vi "M_alpha_beta_2 (SubVI).vi"(4 "i":i32, 6 "Fe_data":dbl[](array[numeric]), 7 "FE [N]":dbl[](array[numeric]), 8 "Vehicle Parameters":T1, 10 "Data":dbl[][](array[numeric]), 11 "cluster":T3) -> (0 "output cluster":T2, 2 "M_beta":dbl, 3 "M_alpha":dbl)   [LabVIEW 2017]
uses:
  <vilib>/Analysis/_algsub.llb/Vector Norm Type.ctl
  <vilib>/Analysis/_algsub.llb/Real Vector Norm.vi
  <vilib>/Analysis/NI_AALPro.lvlib
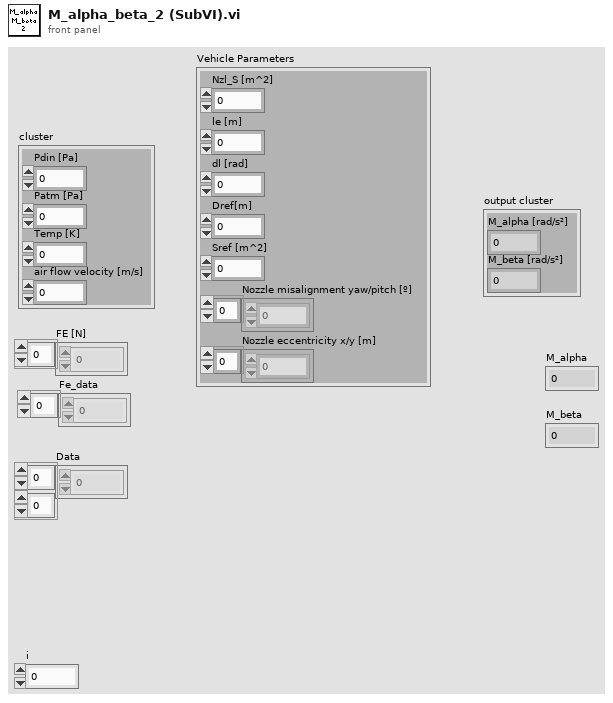
[diagram p1: front panel]
types:
  T1 = cluster{"Nzl_S [m^2]":dbl, "le [m]":dbl, "dl [rad]":dbl, "Dref[m]":dbl, "Sref [m^2]":dbl, "Nozzle misalignment yaw/pitch [º]":dbl[], "Nozzle eccentricity x/y [m]":dbl[]}
  T2 = cluster{"M_alpha [rad/s²]":dbl, "M_beta [rad/s²]":dbl}
  T3 = cluster{"Pdin [Pa]":dbl, "Patm [Pa]":dbl, "Temp [K]":dbl, "air flow velocity [m/s]":dbl}
  T4 = typedef "NI_AALPro.lvlib/Vector Norm Type.ctl" = u16
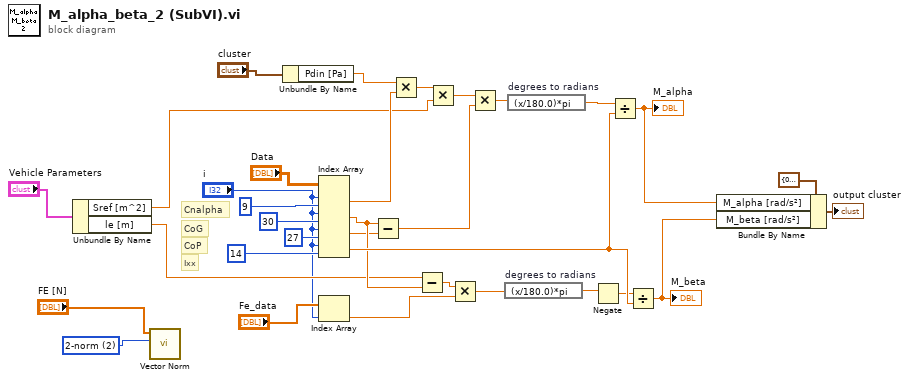
[diagram p0: block diagram]
diagram:
  w26 = T4 2 items=["1-norm"=1, "2-norm"=2, "Inf-norm"=3, "-Inf-norm"=4, "User Defined"=5] ("norm type")
  # "Ixx"
  # "CoP"
  # "CoG"
  # "Cnalpha"
  n1 = Unbundle By Name("Vehicle Parameters") -> ("Sref [m^2]"=w10:dbl, "le [m]"=w11:dbl)
  n2 = call-poly <vilib>:"Vector Norm.vi"("norm type"=w26, "Input Vector"="FE [N]") -> ()  [unwired: 8 in, 2 out]
  n3 = Unbundle By Name("cluster") -> ("Pdin [Pa]"=w13:dbl)
  n4 = Index Array(array="Data", index (row) #1="i", index (col) #1=9 ("disabled index (col)"), index (row) #2="i", index (col) #2=30 ("disabled index (col)"), index (row) #3="i", index (col) #3=27 ("disabled index (col)"), index (row) #4="i", index (col) #4=14 ("disabled index (col)")) -> (element #1=w25:dbl, element #2=w27:dbl, element #3=w20:dbl, element #4=w32:dbl)
  n5 = Index Array(array="Fe_data", index="i") -> (element=w1:dbl)
  n6 = Subtract(x=w27, y=w20) -> (x-y=w22:dbl)
  n7 = Multiply(x=w13, y=w25) -> (x*y=w19:dbl)
  n8 = Subtract(x=w11, y=w27) -> (x-y=w28:dbl)
  n9 = Multiply(x=w19, y=w10) -> (x*y=w21:dbl)
  n10 = Multiply(x=w28, y=w1) -> (x*y=w29:dbl)
  n11 = Multiply(x=w21, y=w22) -> (x*y=w23:dbl)
  n12 = expression code="(x/180.0)*pi" "degrees to radians"(w29) -> (w30:dbl)
  n13 = expression code="(x/180.0)*pi" "degrees to radians"(w23) -> (w24:dbl)
  n14 = Negate(x=w30) -> (-x=w31:dbl)
  n15 = Divide(x=w24, y=w32) -> (x/y=w8:dbl)
  "M_alpha" <- w8
  n16 = Divide(x=w31, y=w32) -> (x/y=w7:dbl)
  "M_beta" <- w7
  n17 = Bundle By Name(cluster=T2 {"M_alpha [rad/s²]"=0.0, "M_beta [rad/s²]"=0.0} ("output cluster 2"), "M_alpha [rad/s²]"=w8, "M_beta [rad/s²]"=w7) -> (→"output cluster":T2)
